vi "4155C Check File Exists.vi"(1 "Path":path) -> (0 "Exists?":bool)   [LabVIEW 2019]
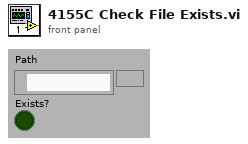
[diagram p1: front panel]
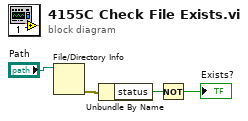
[diagram p0: block diagram]
diagram:
  n1 = File/Directory Info(path="Path") -> (error out=w3:errorcluster)  [unwired: 1 in, 6 out]
  n2 = Unbundle By Name(w3) -> ("status"=w2:bool)
  n3 = Not(x=w2) -> (.not. x?=→"Exists?":bool)
